vi "Query Multi Eval Meas State.vi"(8 "error in (no error)":errorcluster, 10 "Instance (1)":i32=1, 11 "VISA resource name":refnum<visa-resource-name>) -> (0 "error out":errorcluster, 1 "Sync State":i32, 2 "Main State":i32, 3 "VISA resource name out":refnum<visa-resource-name>, 4 "Resources State":i32)   [LabVIEW 2015, in "Rohde&Schwarz CMP LR WPAN Measurement.lvlib"]
doc: "Queries the main measurement state and the measurement substates. Both measurement substates are relevant for running measurements only. Use FETCh:...:STATe? to query the main measurement state only. Use INITiate..., STOP..., ABORt... to change the measurement state.\n\nAttribute:\n-\n\nRemote-control command:\nFETCh:WPAN:MEAS<i>:MEValuation:STATe:ALL?"
uses:
  <instrlib>/Rohde&Schwarz CMP LR WPAN Measurement/Rohde&Schwarz CMP LR WPAN Measurement.lvlib
  <instrlib>/Rohde&Schwarz CMP LR WPAN Measurement/Private/rsidr_core.llb/rsidr_core.lvlib
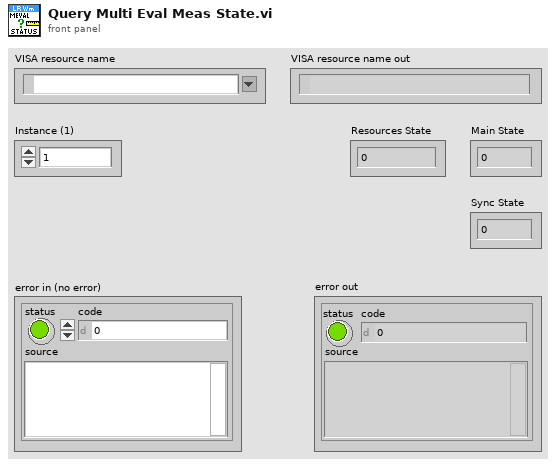
[diagram p1: front panel]
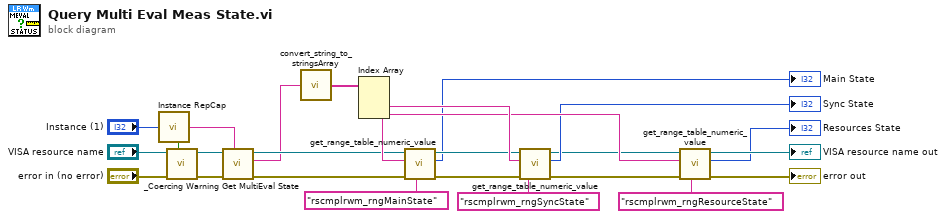
[diagram p0: block diagram]
diagram:
  n1 = call <instrlib>:"Instance RepCap.vi"("Instance In"="Instance (1)") -> ("In Range?"=w26:bool, "RepCap Identifier Out"=w25:string)  [unwired: 1 in]
  n2 = call <instrlib>:"_Coercing Warning.vi"("In Range?"=w26, "error in (no error)"="error in (no error)", "VISA resource name"="VISA resource name") -> ("error out"=w14:errorcluster, "VISA resource name out"=w13:refnum<visa-resource-name>)  [unwired: 7 in]
  n3 = call "Get MultiEval State"("Repeated Capabilities"=w25, "error in (no error)"=w14, "instrument handle"=w13) -> ("error out"=w12:errorcluster, "MultiEval State"=w1:string, "instrument handle out"=w11:refnum<visa-resource-name>)  [unwired: 6 in]
  n4 = call <instrlib>:"convert_string_to_stringsArray.vi"("String in"=w1) -> ("string array out"=w24:string[])  [unwired: 3 in, 1 out]
  n5 = Index Array(array=w24) -> (element #1=w23:string, element #2=w22:string, element #3=w21:string)  [unwired: 3 in]
  n6 = call <instrlib>:"get_range_table_numeric_value.vi"("Range Table ID in"="rscmplrwm_rngMainState", "error in"=w12, "String Value"=w23, "VISA resource name"=w11) -> ("error out"=w10:errorcluster, "I32 output"=→"Main State":i32, "VISA resource name out"=w9:refnum<visa-resource-name>)  [unwired: 5 in]
  n7 = call <instrlib>:"get_range_table_numeric_value.vi"("Range Table ID in"="rscmplrwm_rngSyncState", "error in"=w10, "String Value"=w22, "VISA resource name"=w9) -> ("error out"=w8:errorcluster, "I32 output"=→"Sync State":i32, "VISA resource name out"=w7:refnum<visa-resource-name>)  [unwired: 5 in]
  n8 = call <instrlib>:"get_range_table_numeric_value.vi"("Range Table ID in"="rscmplrwm_rngResourceState", "error in"=w8, "String Value"=w21, "VISA resource name"=w7) -> ("error out"=→"error out":errorcluster, "I32 output"=→"Resources State":i32, "VISA resource name out"=→"VISA resource name out":refnum<visa-resource-name>)  [unwired: 5 in]
